vi "Base settings.vi"(1 "Action(GET)":T3(ring), 7 "Base Setup  In":T1, 11 "error in (no error)":errorcluster) -> (8 "Base Setup Out":T1, 15 "error out":errorcluster)   [LabVIEW 2011]
uses:
  Base settings.ctl
  Program Mode.ctl
  <vilib>/Utility/VariantDataType/VariantType.lvlib
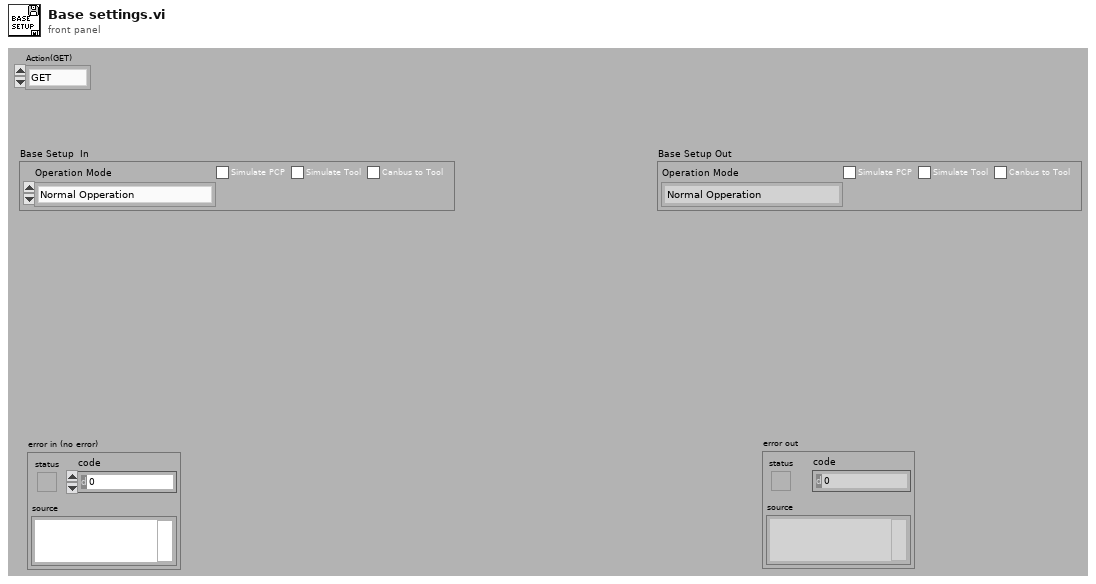
[diagram p1: front panel]
types:
  T1 = typedef "Base settings.ctl" = cluster{"Operation Mode":T2, "Simulate PCP":bool, "Simulate Tool":bool, "Canbus to Tool":bool}
  T2 = typedef "Program Mode.ctl" = enum16{"Normal Opperation", "Setup and Maintenance", "Replay"}
  T3 = enum16{"GET", "SET", "Get from Ini", "Put in Ini"}
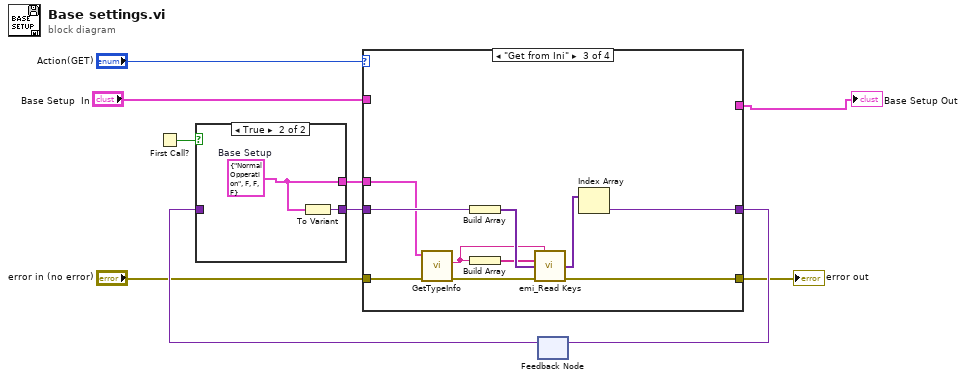
[diagram p0: block diagram]
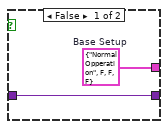
[diagram p2: hidden frame]
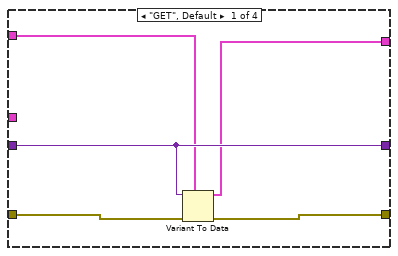
[diagram p3: hidden frame]
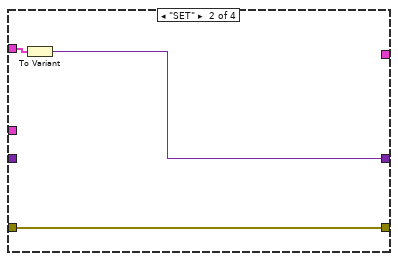
[diagram p4: hidden frame]
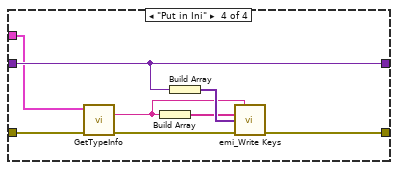
[diagram p5: hidden frame]
diagram:
  n1 = First Call?() -> (First Call?: T/F=w8:bool)
  n2 = feedback #1() -> (w9:variant)  [unwired: 1 in]
  n3 = case shown="True" w8 {
    tunnel: w9 -> [w12 _]
    tunnel: [w12 w14] -> w6
    tunnel: [w11 w13] -> w2
    frame False {
      w11 = T1 {"Operation Mode"=enum."Normal Opperation", "Simulate PCP"=FALSE, "Simulate Tool"=FALSE, "Canbus to Tool"=FALSE}  # Base Setup
    }
    frame True {
      w13 = T1 {"Operation Mode"=enum."Normal Opperation", "Simulate PCP"=FALSE, "Simulate Tool"=FALSE, "Canbus to Tool"=FALSE}  # Base Setup
      n4 = To Variant(anything=w13) -> (Variant=w14:variant)
    }
  }
  n5 = case shown="\"Get from Ini\"" "Action(GET)" {
    tunnel: [w19 w21 w24 w34] -> w7
    tunnel: w6 -> [w19 _ w25 w34]
    tunnel: "error in (no error)" -> [w18 w22 w30 w38]
    tunnel: [w17 w22 w32 w40] -> w4
    tunnel: [w16 _ _ _] -> w1
    tunnel: "Base Setup  In" -> [w15 w20 _ _]
    tunnel: w2 -> [_ _ w23 w33]
    frame "GET", Default {
      n6 = Variant To Data(error in=w18, type=w15, Variant=w19) -> (data=w16:T1, error out=w17:errorcluster)
    }
    frame "SET" {
      n7 = To Variant(anything=w20) -> (Variant=w21:variant)
    }
    frame "Get from Ini" {
      n8 = call <vilib>:"GetTypeInfo.vi"("error in (no error)"=w30, "Variant"=w23) -> ("error out"=w29:errorcluster, "Name"=w27:string)  [unwired: 5 in, 3 out]
      n9 = Build Array(w25) -> (w31:variant[])
      n10 = Build Array(w27) -> (w28:string[])
      n11 = call "emi_Read Keys.vi"("Section"=w27, "Key Names"=w28, "Types/Defaults"=w31, "error in (no error)"=w29) -> ("Values"=w26:variant[], "error out"=w32:errorcluster)  [unwired: 9 in, 1 out]
      n12 = Index Array(array=w26) -> (element=w24:variant)  [unwired: 1 in]
    }
    frame "Put in Ini" {
      n13 = call <vilib>:"GetTypeInfo.vi"("error in (no error)"=w38, "Variant"=w33) -> ("error out"=w37:errorcluster, "Name"=w35:string)  [unwired: 5 in, 3 out]
      n14 = Build Array(w35) -> (w36:string[])
      n15 = Build Array(w34) -> (w39:variant[])
      n16 = call "emi_Write Keys.vi"("Section"=w35, "Key Names"=w36, "Values"=w39, "error in (no error)"=w37) -> ("error out"=w40:errorcluster)  [unwired: 10 in, 1 out]
    }
  }
  "error out" <- w4
  "Base Setup Out" <- w1
  n17 = feedback-in #1(w7) -> ()
